vi "Test-DynamicDependency.vi"() -> ()   [LabVIEW 2013]
uses:
  src/SMO/Typedefs/SMOState --Enum.ctl
  src/SMO/Typedefs/SMO Dependency Event--Enum.ctl
  _test-support-SMOs/SMO.Example/SMO.Example.lvclass
  _test-support-SMOs/SMO.SelfTerminatingOverride/SMO.SelfTerminatingOverride.lvclass
  src/SMO/SMO.lvclass
  src/Registry/Registry-SMO.lvclass
panel:
  in  "Launch Dep 3":bool
  in  "Launch Dep 2":bool
  out "Event":T1
  out "Name":string
  in  "Clear Error":bool
  in  "Stop Dep":bool
  in  "Registered Subsystems":i32(listbox)
  in  "Launch Dep":bool
  out "SMO State":T2
  in  "Stop":bool
  out "error":errorcluster
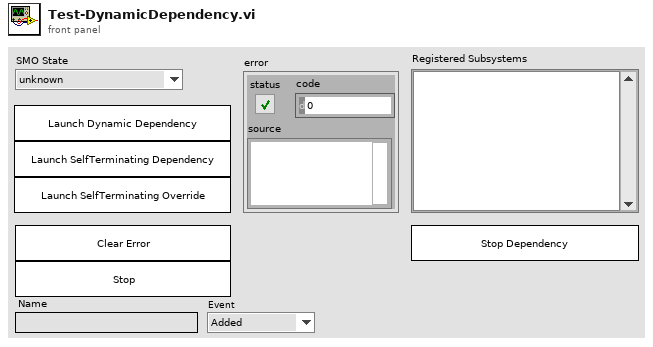
[diagram p1: front panel]
types:
  T1 = typedef "SMO.lvclass/SMO Dependency Event--Enum.ctl" = enum16{"Added", "Removed", "Started", "Stopped"}
  T2 = typedef "SMO.lvclass/SMOState --Enum.ctl" = enum16{"unknown", "Created", "Started", "Stopped"}
  T3 = typedef "Registry-SMO.lvclass/PublicRegistryEvents--Cluster.ctl" = cluster{"Register Event":refnum<user-event>, "Unregister Event":refnum<user-event>}
  T4 = typedef "SMO.lvclass/Public Events.ctl" = cluster{"Error":refnum<user-event>, "State":refnum<user-event>, "Reserve State":refnum<user-event>}
  T5 = cluster{"Event Registration Refnum":refnum<event-registration>}
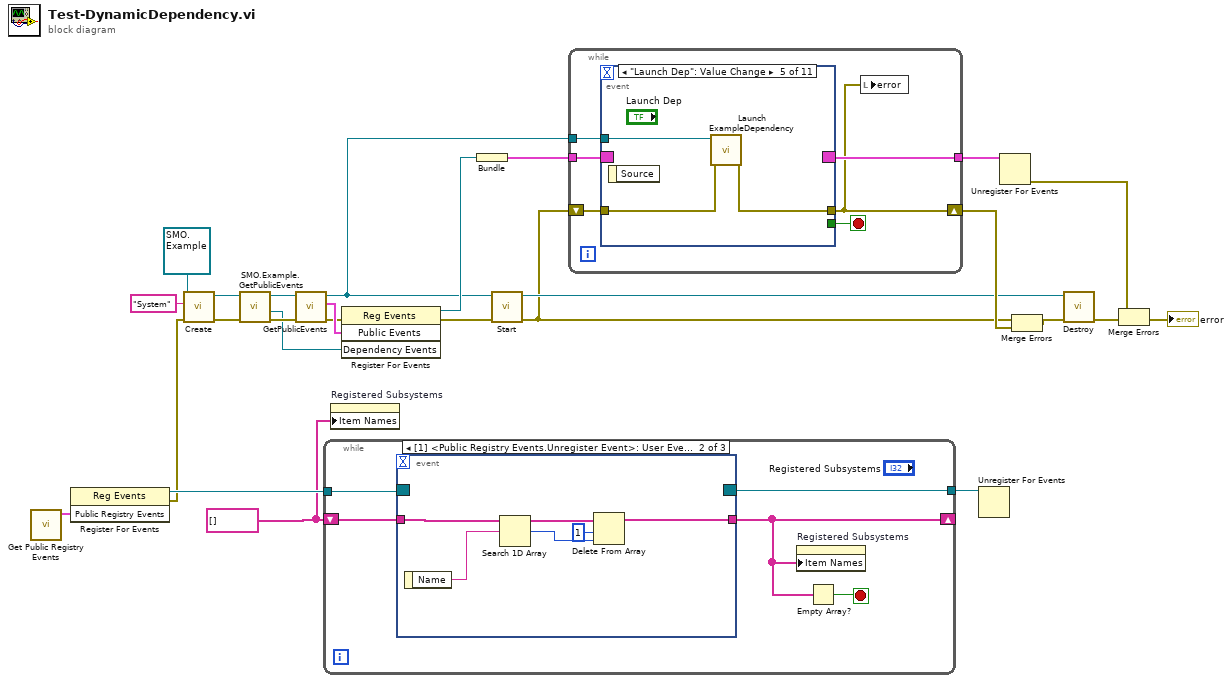
[diagram p0: block diagram]
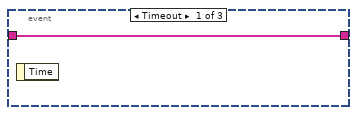
[diagram p2: hidden frame]
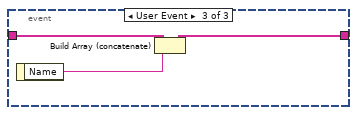
[diagram p3: hidden frame]
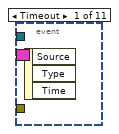
[diagram p4: hidden frame]
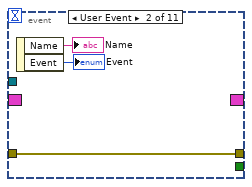
[diagram p5: hidden frame]
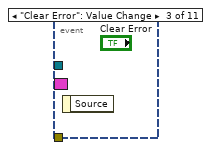
[diagram p6: hidden frame]
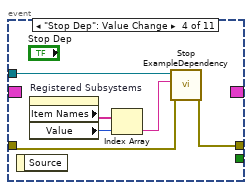
[diagram p7: hidden frame]
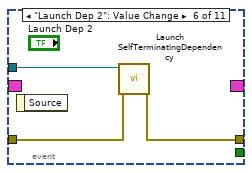
[diagram p8: hidden frame]
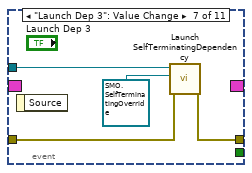
[diagram p9: hidden frame]
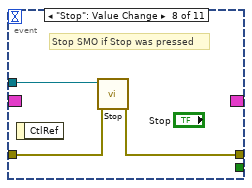
[diagram p10: hidden frame]
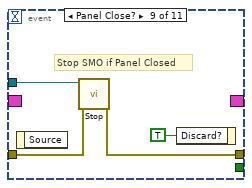
[diagram p11: hidden frame]
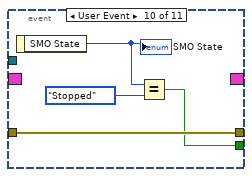
[diagram p12: hidden frame]
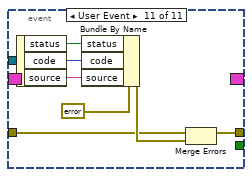
[diagram p13: hidden frame]
diagram:
  w6 = string[] []
  n1 = call "Get Public Registry Events.vi"() -> ("Public Registry Events"=w14:T3)  [unwired: 10 in, 1 out]
  n2 = register-events(w14) -> (reference out=w13:refnum<event-registration>, error out=w12:errorcluster)  [unwired: 2 in]
  n3 = call "Create.vi"("error in (no error)"=w12, "Subsystem Name (optional)"="System", "SMO"=refnum<class "SMO.Example.lvclass"> refnum ("SMO.Example.lvclass")) -> ("error out"=w3:errorcluster, "SMO out"=w5:refnum<class "SMO.Example.lvclass">)  [unwired: 6 in, 1 out]
  n4 = call "SMO.Example.GetPublicEvents.vi"("error in (no error)"=w3, "SMO.Example"=w5) -> ("error out"=w2:errorcluster, "Dependency Events"=w1:refnum<user-event>, "SMO.Example out"=w4:refnum<class "SMO.Example.lvclass">)  [unwired: 6 in, 1 out]
  n5 = call "GetPublicEvents.vi"("error in (no error)"=w2, "SMO"=w4) -> ("error out"=w17:errorcluster, "Public Events"=w19:T4, "SMO out"=w18:refnum<class "SMO.Example.lvclass">)  [unwired: 7 in]
  n6 = while {
    tunnel: w13 -> [w31]
    shift-right: [w27] -> _
    shift-left: w6 -> [w30]
    tunnel: [w28] -> w11
    stop <- w29 stop-if-true
    n7 = event shown="[1] <Public Registry Events.Unregister Event>: User Event" {
      selector: w31 -> [_ _ _]
      dyn-events: [_ _ _] -> w28
      timeout: _ -> [_ _ _]
      tunnel: w30 -> [w32 w36 w40]
      tunnel: [w32 w35 w38] -> w27
      event Timeout {
        n8 = event-data() -> ()  [unwired: 1 in, 1 out]
      }
      event User Event {
        n9 = event-data() -> ("Name"=w37:string)  [unwired: 1 in]
        n10 = Search 1D Array(1D array=w36, element=w37) -> (index of element=w34:i32)  [unwired: 1 in]
        n11 = Delete From Array(array=w36, length=1, index=w34) -> (array with subset deleted=w35:string[])  [unwired: 1 out]
      }
      event User Event {
        n12 = event-data() -> ("Name"=w39:string)  [unwired: 1 in]
        n13 = Build Array (concatenate)(w40, w39) -> (w38:string[])
      }
    }
    n14 = property on="Registered Subsystems" class="LstBox (strict)"("Item Names"=w27) -> ()  [unwired: 2 in, 2 out]
    n15 = Empty Array?(array=w27) -> (empty?=w29:bool)
  }
  n16 = property on="Registered Subsystems" class="LstBox (strict)"("Item Names"=w6) -> ()  [unwired: 2 in, 2 out]
  n17 = register-events(error in=w17, w19, w1) -> (reference out=w21:refnum<event-registration>, error out=w20:errorcluster)  [unwired: 1 in]
  n18 = Bundle("Event Registration Refnum"=w21) -> (w25:T5)  [unwired: 1 in]
  n19 = call "Start.vi"("error in (no error)"=w20, "SMO"=w18) -> ("error out"=w7:errorcluster, "SMO out"=w8:refnum<class "SMO.Example.lvclass">)  [unwired: 8 in]
  n20 = while {
    shift-right: [w41] -> w10
    shift-left: w7 -> [w45]
    tunnel: w25 -> [w44]
    tunnel: [w43] -> w26
    tunnel: w18 -> [w42]
    stop <- w46 stop-if-true
    n21 = event shown="[4] \"Launch Dep\": Value Change" {
      selector: w44 -> [_ _ _ _ _ _ _ _ _ _ _]
      dyn-events: [_ _ _ _ _ _ _ _ _ _ _] -> w43
      timeout: _ -> [_ _ _ _ _ _ _ _ _ _ _]
      tunnel: [_ _ _ _ _ _ _ _ _ w73 _] -> w46
      tunnel: w42 -> [_ _ _ w55 w58 w61 w65 w68 w72 _ _]
      tunnel: [_ w47 _ w53 w56 w59 w63 w67 w71 w74 w77] -> w41
      tunnel: w45 -> [_ w47 _ w54 w57 w60 w64 w66 w70 w74 w78]
      event Timeout {
        n22 = event-data() -> ()  [unwired: 1 in, 3 out]
      }
      event User Event {
        n23 = event-data() -> ("Name"=→"Name":string, "Event"=→"Event":T1)  [unwired: 1 in]
      }
      event "Clear Error": Value Change {
        n24 = event-data() -> ()  [unwired: 1 in, 1 out]
      }
      event "Stop Dep": Value Change {
        n25 = event-data() -> ()  [unwired: 1 in, 1 out]
        n26 = property on="Registered Subsystems" class="LstBox (strict)"() -> ("Item Names"=w52:string[], "Value"=w51:i32)  [unwired: 2 in, 2 out]
        n27 = Index Array(array=w52, index=w51) -> (element=w50:string)
        n28 = call "Stop ExampleDependency.vi"("error in (no error)"=w54, "Dependency Name"=w50, "SMO.Example in"=w55) -> ("error out"=w53:errorcluster)  [unwired: 7 in, 1 out]
      }
      event "Launch Dep": Value Change {
        n29 = event-data() -> ()  [unwired: 1 in, 1 out]
        n30 = call "Launch ExampleDependency.vi"("error in (no error)"=w57, "SMO.Example in"=w58) -> ("error out"=w56:errorcluster)  [unwired: 6 in, 3 out]
      }
      event "Launch Dep 2": Value Change {
        n31 = event-data() -> ()  [unwired: 1 in, 1 out]
        n32 = call "Launch SelfTerminatingDependency.vi"("error in (no error)"=w60, "SMO.Example in"=w61) -> ("error out"=w59:errorcluster)  [unwired: 8 in, 1 out]
      }
      event "Launch Dep 3": Value Change {
        n33 = event-data() -> ()  [unwired: 1 in, 1 out]
        n34 = call "Launch SelfTerminatingDependency.vi"("error in (no error)"=w64, "SMO.SelfTerminating type"=refnum<class "SMO.SelfTerminatingOverride.lvclass"> refnum ("SMO.SelfTerminatingOverride.lvclass"), "SMO.Example in"=w65) -> ("error out"=w63:errorcluster)  [unwired: 7 in, 1 out]
      }
      event "Stop": Value Change {
        # "Stop SMO if Stop was pressed"
        n35 = event-data() -> ()  [unwired: 1 in, 1 out]
        n36 = call "Stop.vi"("error in (no error)"=w66, "SMO"=w68) -> ("error out"=w67:errorcluster)  [unwired: 8 in, 1 out]
      }
      event Panel Close? {
        # "Stop SMO if Panel Closed"
        n37 = event-data() -> ()  [unwired: 1 in, 1 out]
        n38 = call "Stop.vi"("error in (no error)"=w70, "SMO"=w72) -> ("error out"=w71:errorcluster)  [unwired: 8 in, 1 out]
        n39 = event-data("Discard?"=TRUE ("OK")) -> ()  [unwired: 1 in, 1 out]
      }
      event User Event {
        n40 = event-data() -> ("SMO State"=w76:T2)  [unwired: 1 in]
        "SMO State" <- w76
        n41 = Equal?(x=w76, y=SMOState_--Enum."Stopped") -> (x = y?=w73:bool)
      }
      event User Event {
        n42 = event-data() -> ("status"=w83:bool, "code"=w81:i32, "source"=w80:string)  [unwired: 1 in]
        n43 = Bundle By Name(cluster=errorcluster {"status"=FALSE, "code"=0, "source"=""} ("error constant"), "status"=w83, "code"=w81, "source"=w80) -> (w79:errorcluster)
        n44 = Merge Errors(w78, w79) -> (w77:errorcluster)
      }
    }
    n45 = local write "error"(w41) -> ()
  }
  n46 = Unregister For Events(event registration refnum=w11) -> ()  [unwired: 1 in, 1 out]
  n47 = Unregister For Events(event registration refnum=w26) -> (error out=w24:errorcluster)  [unwired: 1 in]
  n48 = Merge Errors(w7, w10) -> (w16:errorcluster)
  n49 = call "Destroy.vi"("error in (no error)"=w16, "SMO"=w8) -> ("error out"=w22:errorcluster)  [unwired: 9 in]
  n50 = Merge Errors(w24, w22) -> (→"error":errorcluster)
